vi "Begin.vi"(8 "error in":errorcluster) -> (0 "error out":errorcluster)   [LabVIEW 2018]
doc: "Called before other user functions, this VI is expected to open initial I/O refnums, load in file data, and do all program initialization. Notice that the <B>error out</B> terminal is simply used for data flow. Wiring it to other structures or subVIs ensures that this VI runs first."
uses:
  <vilib>/Rock Robotics/SystemInterfaces/DIO/FPGA_DIOPWMChannel.ctl
  <vilib>/Rock Robotics/WPI/SafetyOutput/WPI_SafetyOutputConfigMenu.ctl
  <vilib>/Rock Robotics/WPI/DriverStation/WPI_DriverStationRobotMode2.ctl
  <vilib>/Rock Robotics/WPI/Joystick/WPI_JoystickDeviceEnum.ctl
  <vilib>/Rock Robotics/WPI/Solenoid/WPI_SolenoidChannel.ctl
  Robot Global Data.vi
  <vilib>/Rock Robotics/Network Tables/NT Write String Array.vi
  <vilib>/Rock Robotics/WPI/RobotDrive/WPI_RobotDriveOpen4MotorWithSPARK.vi
  <vilib>/Rock Robotics/WPI/Utilities/WPI_GetSetVariantRefNum.vi
  <vilib>/Rock Robotics/WPI/Solenoid/WPI_SolenoidOpenDouble.vi
  <vilib>/Rock Robotics/WPI/MotorControl/WPI_MotorControlOpen SPARK.vi
  <vilib>/Rock Robotics/WPI/Gyro/WPI_GyroAnalogOpen.vi
  <vilib>/Rock Robotics/SystemInterfaces/spilib/spi_bus.ctl
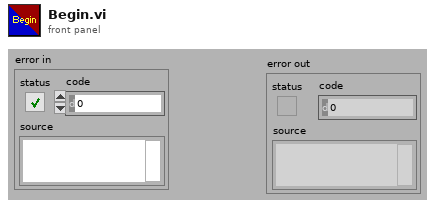
[diagram p1: front panel]
types:
  T1 = typedef "FPGA_DIOPWMChannel.ctl" = enum8{"PWM 0", "PWM 1", "PWM 2", "PWM 3", "PWM 4", "PWM 5", "PWM 6", "PWM 7", "PWM 8", "PWM 9", "PWM MXP 0", "PWM MXP 1", "PWM MXP 2", "PWM MXP 3", "PWM MXP 4", "PWM MXP 5", "PWM MXP 6", "PWM MXP 7", "PWM MXP 8", "PWM MXP 9", "Invalid"}
  T2 = typedef "WPI_SolenoidChannel.ctl" = enum8{"Solenoid 0", "Solenoid 1", "Solenoid 2", "Solenoid 3", "Solenoid 4", "Solenoid 5", "Solenoid 6", "Solenoid 7", "Invalid"}
  T3 = typedef "WPI_JoystickDeviceEnum.ctl" = enum16{"USB 0", "USB 1", "USB 2", "USB 3", "USB 4", "USB 5"}
  T4 = typedef "WPI_DriverStationRobotMode2.ctl" = enum16{"Autonomous Disabled", "Autonomous Enabled", "Teleop Disabled", "Teleop Enabled", "Disconnected", "Finish", "Test Disabled", "Test Enabled", "Emergency Stopped"}
  T5 = typedef "WPI_SafetyOutputConfigMenu.ctl" = enum16{"Enable", "Disable"}
  T6 = typedef "WPI_CompressorDevRef.ctl" = cluster{"DevStatus":errorcluster, "Pneumatics Control Module":u8}
  T7 = typedef "WPI_MotorControlDeviceRef.ctl" = cluster{"DeviceStatus":errorcluster, "Type":T8, "PWM":cluster{"PWM Channel":T1, "DeadBand":T9}, "CAN":cluster{"Device Number":u8, "SetOutput VI Ref":variant, "GetOutput VI Ref":variant, "Enable VI Ref":variant, "Disable VI Ref":variant, "Data":variant}, "Invert":bool, "DIO PWM":cluster{"PWM \"Enable\" Channel":T1, "DIOChannel":T10, "PWM Rate":dbl}}
  T8 = typedef "WPI_MotorControlType.ctl" = enum16{"PWM", "CAN", "DIO PWM"}
  T9 = typedef "WPI_PWMDeadband.ctl" = cluster{"Name":string, "maxPositivePwm":i32, "minPositivePwm":i32, "centerPwm":i32, "maxNegativePwm":i32, "minNegativePwm":i32, "angularRange":u16}
  T10 = typedef "FPGA_DIOChannel.ctl" = enum8{"DIO 0", "DIO 1", "DIO 2", "DIO 3", "DIO 4", "DIO 5", "DIO 6", "DIO 7", "DIO 8", "DIO 9", "DIO MXP 0", "DIO MXP 1", "DIO MXP 2", "DIO MXP 3", "DIO MXP 4", "DIO MXP 5", "DIO MXP 6", "DIO MXP 7", "DIO MXP 8", "DIO MXP 9", "DIO MXP 10", "DIO MXP 11", "DIO MXP 12", "DIO MXP 13", "DIO MXP 14", "DIO MXP 15", "SPI Port CS1", "SPI Port CS2", "SPI Port CS3", "SPI Port MISO", "SPI Port MOSI", "Invalid"}
  T11 = typedef "WPI_JoystickDevRef.ctl" = cluster{"Device":T3}
  T12 = typedef "WPI_SolenoidDevRef.ctl" = cluster{"DevStatus":errorcluster, "Pneumatics Control Module":u8, "Forward Solenoid Channel":T2, "Reverse Solenoid Channel":T2}
  T13 = typedef "WPI_RobotDriveDevRef.ctl" = cluster{"DevStatus":errorcluster, "Motors[]":T7[], "Square Inputs":bool, "Max Output":dbl}
  T14 = typedef "spi_bus.ctl" = enum16{"SPI On-Board, CS0", "SPI On-Board, CS1", "SPI On-Board, CS2", "SPI On-Board, CS3", "SPI MXP", "Invalid"}
  T15 = typedef "WPI_GyroDevRef.ctl" = cluster{"DevStatus":errorcluster, "Analog Channel":T16, "Gain (VoltsPerDegree/Second)":dbl, "Gyro Type":enum16{"Analog", "XRS450"}, "Handle":i32, "SPI Bus":T14, "Device Found":bool, "Sample Rate":dbl, "Calibrate On Open":bool, "Offset":dbl}
  T16 = typedef "FPGA_AIChannel.ctl" = enum8{"AI 0", "AI 1", "AI 2", "AI 3", "AI MXP 0", "AI MXP 1", "AI MXP 2", "AI MXP 3", "Invalid"}
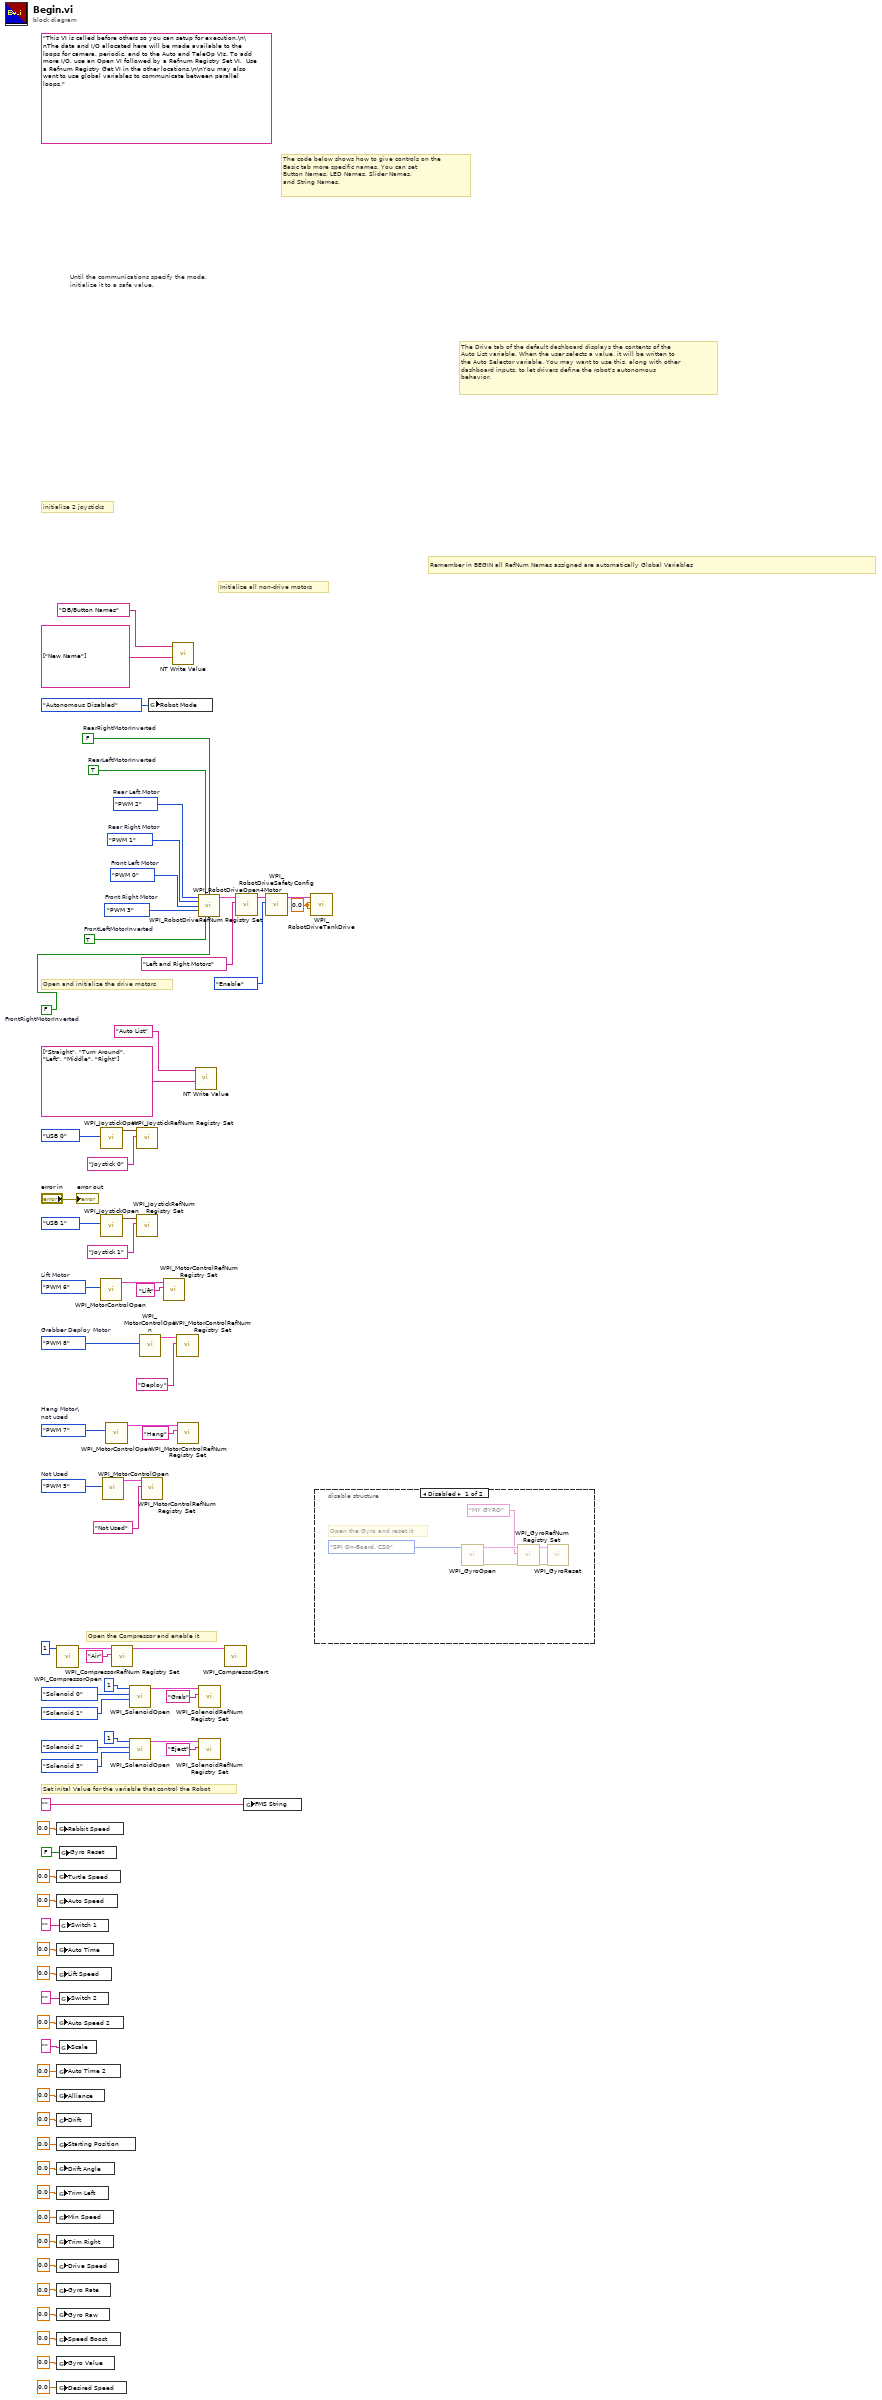
[diagram p0: block diagram]
diagram:
  w1 = FPGA_DIOPWMChannel."PWM 7"  # Hang Motor\ not used
  w4 = FPGA_DIOPWMChannel."PWM 8"  # Grabber Deploy Motor
  w7 = FPGA_DIOPWMChannel."PWM 6"  # Lift Motor
  w11 = FPGA_DIOPWMChannel."PWM 5"  # Not Used
  w22 = 0.0 ("Left axis value")
  w57 = FALSE  # FrontRightMotorInverted
  w58 = TRUE  # FrontLeftMotorInverted
  w61 = FPGA_DIOPWMChannel."PWM 3"  # Front Right Motor
  w62 = FPGA_DIOPWMChannel."PWM 0"  # Front Left Motor
  (unwired) "This VI is called before others so you can setup for execution.\n\nThe data and I/O allocated here will be made available to the loops for camera, periodic, and to the Auto and TeleOp VIs. To add more I/O, use an Open VI followed by a Refnum Registry Set VI.  Use a Refnum Registry Get VI in the other locations.\n\nYou may also want to use global variables to communicate between parallel loops."
  w63 = FPGA_DIOPWMChannel."PWM 1"  # Rear Right Motor
  w64 = FPGA_DIOPWMChannel."PWM 2"  # Rear Left Motor
  w59 = TRUE  # RearLeftMotorInverted
  w60 = FALSE  # RearRightMotorInverted
  # "Initialize all non-drive motors"
  # "Set inital Value for the variable that control the Robot"
  # "Open and initialize the drive motors"
  # "Remember in BEGIN all RefNum Names assigned are automatically Global Variables"
  # "Open the Compressor and enable it"
  # "The Drive tab of the default dashboard displays the contents of the\nAuto List variable. When the user selects a value, it will be written to\nthe Auto Selector variable. You may want to use this, along with other\ndashboard inputs, to let drivers define the robot's autonomous\nbehavior."
  # "The code below shows how to give controls on the\nBasic tab more specific names. You can set\nButton Names, LED Names, Slider Names,\nand String Names."
  # "initialize 2 joysticks"
  # "Until the communications specify the mode,\ninitialize it to a safe value."
  n1 = call <vilib>:"WPI_CompressorOpen.vi"("Pneumatics Control Module (0)"=u8 1) -> ("CompressorDevRef"=w53:T6)  [unwired: 13 in, 1 out]
  n2 = global write "Robot Global Data.vi" "Rabbit Speed"(0.0 ("Alliance")) -> ()
  n3 = global write "Robot Global Data.vi" "Turtle Speed"(0.0 ("Alliance")) -> ()
  n4 = global write "Robot Global Data.vi" "Auto Speed"(0.0 ("Auto Speed")) -> ()
  n5 = global write "Robot Global Data.vi" "Auto Time"(0.0 ("Auto Time")) -> ()
  n6 = global write "Robot Global Data.vi" "Lift Speed"(0.0 ("Alliance")) -> ()
  n7 = global write "Robot Global Data.vi" "Auto Speed 2"(0.0 ("Auto Speed")) -> ()
  n8 = global write "Robot Global Data.vi" "Auto Time 2"(0.0 ("Auto Time")) -> ()
  n9 = global write "Robot Global Data.vi" "Alliance"(0.0 ("Alliance")) -> ()
  n10 = global write "Robot Global Data.vi" "Drift"(0.0 ("Drift")) -> ()
  n11 = global write "Robot Global Data.vi" "Starting Position"(0.0 ("Starting Position")) -> ()
  n12 = global write "Robot Global Data.vi" "Drift Angle"(0.0 ("Drift")) -> ()
  n13 = global write "Robot Global Data.vi" "Trim Left"(0.0 ("Alliance")) -> ()
  n14 = global write "Robot Global Data.vi" "Min Speed"(0.0 ("Alliance")) -> ()
  n15 = global write "Robot Global Data.vi" "Trim Right"(0.0 ("Alliance")) -> ()
  n16 = global write "Robot Global Data.vi" "Drive Speed"(0.0 ("Alliance")) -> ()
  n17 = global write "Robot Global Data.vi" "Gyro Rate"(0.0 ("Alliance")) -> ()
  n18 = global write "Robot Global Data.vi" "Gyro Raw"(0.0 ("Alliance")) -> ()
  n19 = global write "Robot Global Data.vi" "Speed Boost"(0.0 ("Alliance")) -> ()
  n20 = global write "Robot Global Data.vi" "Gyro Value"(0.0 ("Alliance")) -> ()
  n21 = global write "Robot Global Data.vi" "Desired Speed"(0.0 ("Alliance")) -> ()
  n22 = global write "Robot Global Data.vi" "Gyro Reset"(FALSE ("Gyro Reset")) -> ()
  n23 = global write "Robot Global Data.vi" "Switch 1"("" ("Switch 1")) -> ()
  n24 = global write "Robot Global Data.vi" "Switch 2"("" ("Switch 2")) -> ()
  n25 = global write "Robot Global Data.vi" "Scale"("" ("Scale")) -> ()
  n26 = call-poly <vilib>:"WPI_MotorControlOpen.vi"("PWM Channel"=w7) -> ("MotorControlDeviceRef"=w9:T7)  [unwired: 9 in, 1 out]
  n27 = call <vilib>:"WPI_JoystickOpen.vi"("JoystickDevice"=WPI_JoystickDeviceEnum."USB 0") -> ("JoystickDevRef"=w72:T11)  [unwired: 10 in]
  n28 = call <vilib>:"WPI_JoystickOpen.vi"("JoystickDevice"=WPI_JoystickDeviceEnum."USB 1") -> ("JoystickDevRef"=w55:T11)  [unwired: 10 in]
  n29 = call-poly <vilib>:"WPI_MotorControlOpen.vi"("PWM Channel"=w11) -> ("MotorControlDeviceRef"=w12:T7)  [unwired: 9 in, 1 out]
  n30 = call-poly <vilib>:"WPI_MotorControlOpen.vi"("PWM Channel"=w1) -> ("MotorControlDeviceRef"=w3:T7)  [unwired: 9 in, 1 out]
  n31 = call <vilib>:"WPI_CompressorRefNum Registry Set.vi"("refnum name"="Air", "CompressorDevRef"=w53) -> ("CompressorDevRef"=w51:T6)  [unwired: 8 in, 1 out]
  n32 = call-poly <vilib>:"WPI_SolenoidOpen.vi"("Reverse Solenoid Channel"=WPI_SolenoidChannel."Solenoid 1", "Forward Solenoid Channel"=WPI_SolenoidChannel."Solenoid 0", "Pneumatics Control Module (0)"=u8 1) -> ("SolenoidDevRef"=w28:T12)  [unwired: 7 in, 1 out]
  n33 = call-poly <vilib>:"WPI_SolenoidOpen.vi"("Reverse Solenoid Channel"=WPI_SolenoidChannel."Solenoid 3", "Forward Solenoid Channel"=WPI_SolenoidChannel."Solenoid 2", "Pneumatics Control Module (0)"=u8 1) -> ("SolenoidDevRef"=w35:T12)  [unwired: 7 in, 1 out]
  n34 = call <vilib>:"WPI_JoystickRefNum Registry Set.vi"("refnum name"="Joystick 0", "JoystickDevRef"=w72) -> ()  [unwired: 8 in, 2 out]
  n35 = call <vilib>:"WPI_JoystickRefNum Registry Set.vi"("refnum name"="Joystick 1", "JoystickDevRef"=w55) -> ()  [unwired: 8 in, 2 out]
  n36 = call-poly <vilib>:"WPI_MotorControlOpen.vi"("PWM Channel"=w4) -> ("MotorControlDeviceRef"=w6:T7)  [unwired: 9 in, 1 out]
  n37 = call <vilib>:"WPI_MotorControlRefNum Registry Set.vi"("refnum name"="Not Used", "MotorControlDevRef"=w12) -> ()  [unwired: 8 in, 2 out]
  n38 = global write "Robot Global Data.vi" "Robot Mode"(WPI_DriverStationRobotMode2."Autonomous Disabled" ("Robot Mode")) -> ()
  n39 = call <vilib>:"WPI_MotorControlRefNum Registry Set.vi"("refnum name"="Lift", "MotorControlDevRef"=w9) -> ()  [unwired: 8 in, 2 out]
  n40 = call-poly <vilib>:"NT Write Value.vi"("String Array"=string[] ["New Name"], "Name"="DB/Button Names") -> ()  [unwired: 9 in, 1 out]
  n41 = call <vilib>:"WPI_MotorControlRefNum Registry Set.vi"("refnum name"="Deploy", "MotorControlDevRef"=w6) -> ()  [unwired: 8 in, 2 out]
  n42 = call <vilib>:"WPI_MotorControlRefNum Registry Set.vi"("refnum name"="Hang", "MotorControlDevRef"=w3) -> ()  [unwired: 8 in, 2 out]
  n43 = call-poly <vilib>:"NT Write Value.vi"("String Array"=string[] ["Straight", "Turn Around", "Left", "Middle", "Right"], "Name"="Auto List") -> ()  [unwired: 9 in, 1 out]
  n44 = call-poly <vilib>:"WPI_RobotDriveOpen4Motor.vi"("Rear Left Motor"=w64, "Rear Left Motor Inverted"=w59, "Rear Right Motor Inverted"=w60, "Rear Right Motor"=w63, "Front Left Motor"=w62, "Front Right Motor"=w61, "Front Left Motor Inverted"=w58, "Front Right Motor Inverted"=w57) -> ("RobotDriveDevRef"=w65:T13)  [unwired: 6 in, 1 out]
  n45 = call <vilib>:"WPI_SolenoidRefNum Registry Set.vi"("refnum name"="Grab", "SolenoidDevRef"=w28) -> ()  [unwired: 8 in, 2 out]
  n46 = call <vilib>:"WPI_SolenoidRefNum Registry Set.vi"("refnum name"="Eject", "SolenoidDevRef"=w35) -> ()  [unwired: 8 in, 2 out]
  n47 = call <vilib>:"WPI_CompressorStart.vi"("CompressorDevRef"=w51) -> ()  [unwired: 9 in, 2 out]
  n48 = call <vilib>:"WPI_RobotDriveRefNum Registry Set.vi"("refnum name"="Left and Right Motors", "RobotDriveDevRef"=w65) -> ("RobotDriveDevRef"=w76:T13)  [unwired: 2 in, 7 out]
  n49 = global write "Robot Global Data.vi" "FMS String"("" ("FMS String")) -> ()
  n50 = call <vilib>:"WPI_RobotDriveSafetyConfig.vi"("mode"=WPI_SafetyOutputConfigMenu."Enable", "RobotDriveDevRef"=w76) -> ("RobotDriveDevRef"=w23:T13)  [unwired: 8 in, 1 out]
  n51 = call <vilib>:"WPI_RobotDriveTankDrive.vi"("Right axis value"=w22, "Left axis value"=w22, "RobotDriveDevRef"=w23) -> ()  [unwired: 6 in, 3 out]
  n52 = disable-structure shown="Disabled" {
    frame Disabled {
      # "Open the Gyro and reset it"
      n53 = call-poly <vilib>:"WPI_GyroOpen.vi"(11:spi_bus."SPI On-Board, CS0" ("SPI Bus")) -> ("error out"=w83:errorcluster, "GyroDevRef"=w82:T15)  [unwired: 8 in, 1 out]
      n54 = call <vilib>:"WPI_GyroRefNum Registry Set.vi"("error in (no error)"=w83, "refnum name"="MY GYRO", "GyroDevRef"=w82) -> ("error out"=w78:errorcluster, "GyroDevRef"=w79:T15)  [unwired: 7 in]
      n55 = call <vilib>:"WPI_GyroReset.vi"("error in"=w78, "GyroDevRef"=w79) -> ()  [unwired: 8 in, 2 out]
    }
    frame Enabled {
    }
  }
  "error out" <- "error in"
